vi "TestArmPathPlanner.vi"() -> ()   [LabVIEW 2017]
uses:
  General/PathPlanning/TypeDefs/Point2D.ctl
  General/MotionProfiling/TypeDefs/MotionProfileGeneratorParams.ctl
  <vilib>/Rock Robotics/WPI/ThirdParty/Phoenix-LabVIEW/Motor Controller/Controls/CTRE_Phoenix_MotorControl_TrajectoryPointTimeDur.ctl
  General/MotionProfiling/TypeDefs/TrajectoryPoint.ctl
panel:
  out "Arm Rotation":T1(graph)
  out "Arm Extension":T1(graph)
  out "Overall Motion":T1(graph)
  out "TravelTime (s)":dbl
  in  "MotionProfileGeneratorParameters":T2={"Trajectory Point Interval (ms)"=10, "Maximum Travel Speed (rpm)"=5000.0, "Velocity Ramp Time (ms)"=500.0, "Acceleration Ramp Time (ms)"=200.0} {"Acceleration Ramp Time (ms)" min=1.0; "Velocity Ramp Time (ms)" min=1.0; "Maximum Travel Speed (rpm)" min=0.0; "Trajectory Point Interval (ms)" items=["TrajectoryDuration_0ms"=0, "TrajectoryDuration_5ms"=5, "TrajectoryDuration_10ms"=10, "TrajectoryDuration_20ms"=20, "TrajectoryDuration_30ms"=30, "TrajectoryDuration_40ms"=40, "TrajectoryDuration_50ms"=50, "TrajectoryDuration_100ms"=100]}
  in  "EndPoint":T4={"X"=30.0, "Y"=30.0}
  in  "StartPoint":T4={"X"=30.0, "Y"=-24.0}
  in  "PathPointSpacing (in)":dbl=0.25
  in  "MaxArmLength":dbl=48.0
  in  "MinArmLength":dbl=24.0
  out "PathLength (in)":dbl
  out "NumPoints":i32
  out "Path":cluster{dbl[], dbl[]}[](graph)
  out "Update Rate (Hz)":dbl
  in  "stop":bool
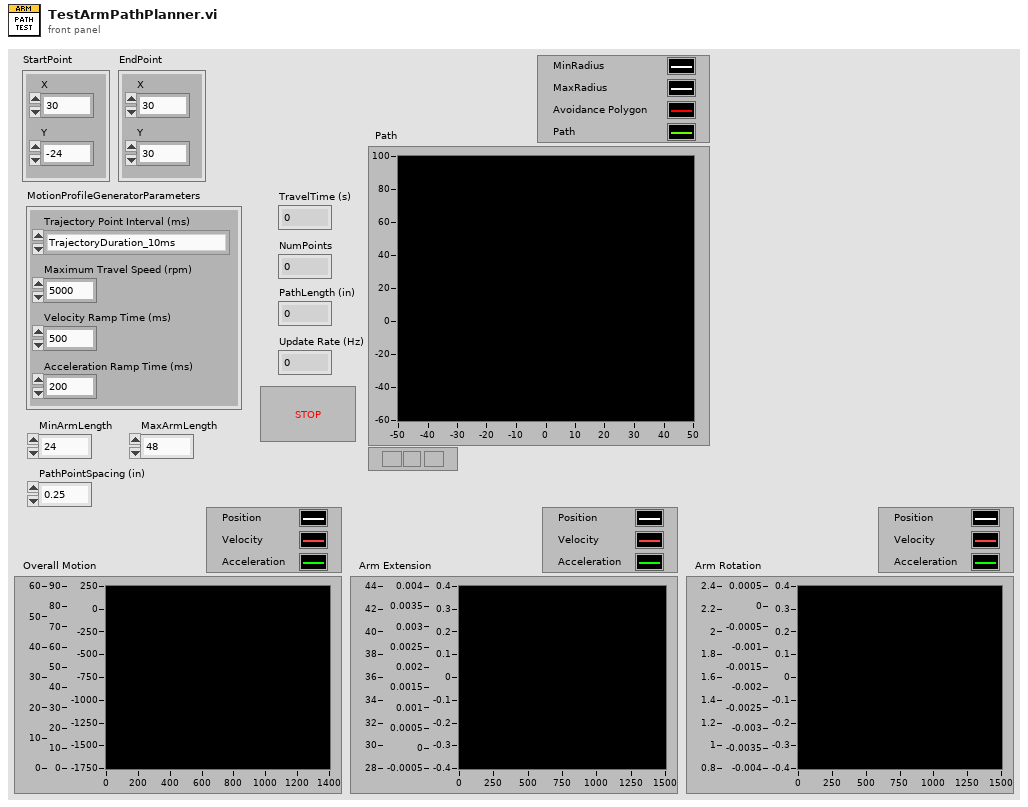
[diagram p1: front panel]
types:
  T1 = cluster{dbl, "Trajectory Point Interval (ms)":i32, dbl[][]}
  T2 = typedef "MotionProfileGeneratorParams.ctl" = cluster{"Trajectory Point Interval (ms)":T3, "Maximum Travel Speed (rpm)":dbl, "Velocity Ramp Time (ms)":dbl, "Acceleration Ramp Time (ms)":dbl}
  T3 = typedef "CTRE_Phoenix_MotorControl_TrajectoryPointTimeDur.ctl" = i32
  T4 = typedef "Point2D.ctl" = cluster{"X":dbl, "Y":dbl}
  T5 = typedef "TrajectoryPoint.ctl" = cluster{"Position ":dbl, "Velocity ":dbl, "Time (ms)":T3, "Last Point":bool}
  T6 = typedef "ArmCoordinate.ctl" = cluster{"Radius (in)":dbl, "Angle (rad)":dbl}
  T7 = cluster{dbl, "Trajectory Point Interval (ms)":T3, dbl[][]}
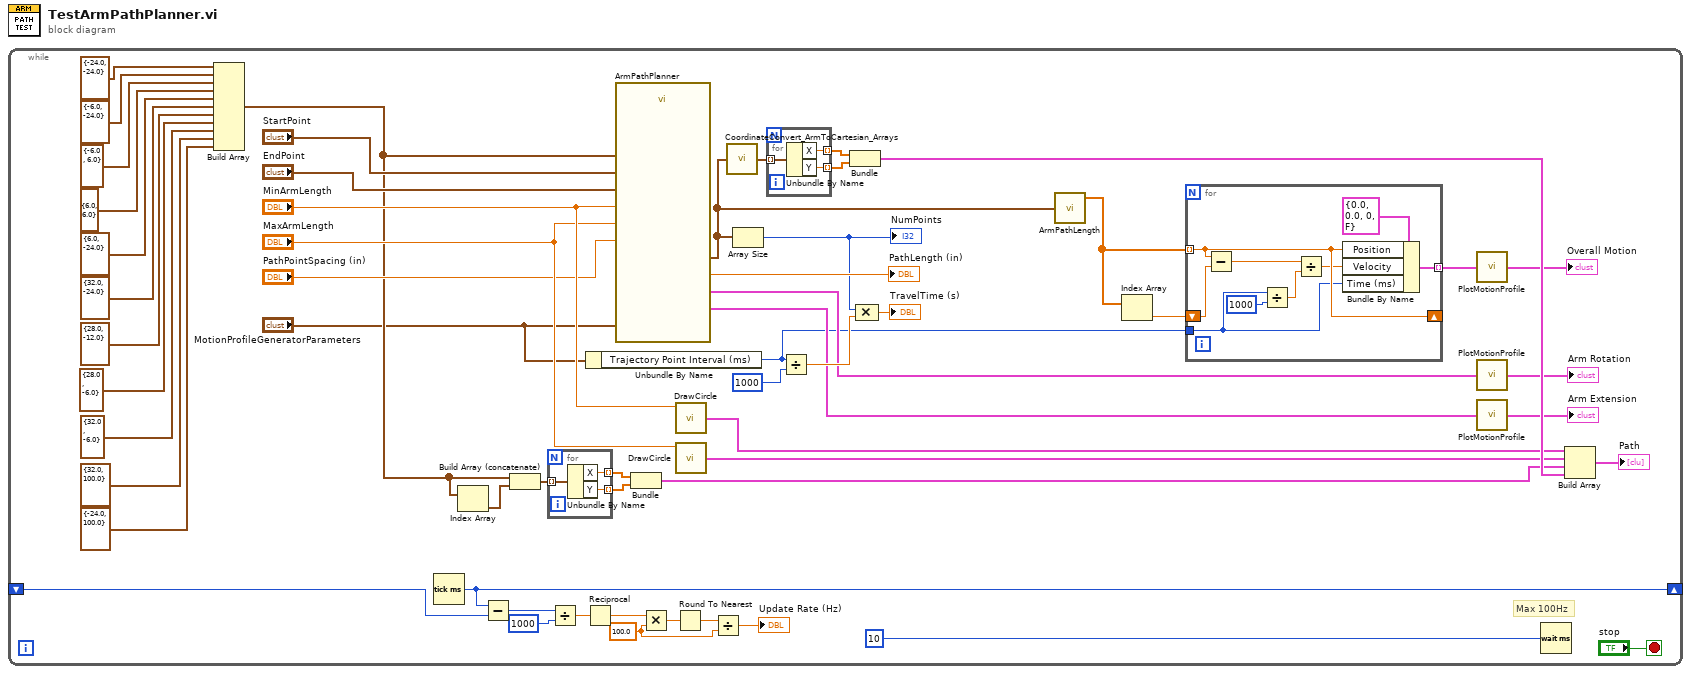
[diagram p0: block diagram]
diagram:
  n1 = while {
    shift-right: [w47] -> _
    shift-left: _ -> [w48]
    stop <- "stop" stop-if-true
    w50 = 100.0 ("y")
    # "Max 100Hz"
    n2 = Build Array(T4 {"X"=-24.0, "Y"=-24.0} ("2DPoint"), T4 {"X"=-6.0, "Y"=-24.0} ("2DPoint"), T4 {"X"=-6.0, "Y"=6.0} ("2DPoint"), T4 {"X"=6.0, "Y"=6.0} ("2DPoint"), T4 {"X"=6.0, "Y"=-24.0} ("2DPoint"), T4 {"X"=32.0, "Y"=-24.0} ("2DPoint"), T4 {"X"=28.0, "Y"=-12.0} ("2DPoint"), T4 {"X"=28.0, "Y"=-6.0} ("2DPoint"), T4 {"X"=32.0, "Y"=-6.0} ("2DPoint"), T4 {"X"=32.0, "Y"=100.0} ("2DPoint"), T4 {"X"=-24.0, "Y"=100.0} ("2DPoint")) -> (w16:T4[])
    n3 = Tick Count (ms)() -> (millisecond timer value=w47:u32)
    n4 = Index Array(array=w16) -> (element=w22:T4)  [unwired: 1 in]
    n5 = Subtract(x=w47, y=w48) -> (x-y=w56:u32)
    n6 = Build Array (concatenate)(w16, w22) -> (w23:T4[])
    n7 = for {
      tunnel: w23 -> [w69] mode=indexing
      tunnel: [w68] -> w38 mode=indexing
      tunnel: [w67] -> w39 mode=indexing
      n8 = Unbundle By Name(w69) -> ("X"=w68:dbl, "Y"=w67:dbl)
    }
    n9 = Divide(x=w56, y=u32 1000) -> (x/y=w54:dbl)
    n10 = Reciprocal(x=w54) -> (1/x=w53:dbl)
    n11 = Unbundle By Name("MotionProfileGeneratorParameters") -> ("Trajectory Point Interval (ms)"=w3:T3)
    n12 = call "ArmPathPlanner.vi"("StartPoint"="StartPoint", "EndPoint"="EndPoint", "PathPointSpacing (in)"="PathPointSpacing (in)", "MinArmLength"="MinArmLength", "MaxArmLength"="MaxArmLength", "AvoidancePolygon"=w16, "MotionProfileGeneratorParameters"="MotionProfileGeneratorParameters") -> ("Path"=w4:T6[], "RotatePath"=w8:T5[], "ExtendPath"=w7:T5[], "PathLength (in)"=→"PathLength (in)":dbl)  [unwired: 9 in]
    n13 = Bundle(w38, w39) -> (w37:cluster{dbl[], dbl[]})  [unwired: 1 in]
    n14 = Multiply(x=w53, y=w50) -> (x*y=w52:dbl)
    n15 = Round To Nearest(number=w52) -> (nearest integer value=w51:dbl)
    n16 = call "DrawCircle.vi"("Radius"="MinArmLength") -> ("Points"=w35:cluster{"X":dbl[], "Y":dbl[]})  [unwired: 3 in]
    n17 = call "DrawCircle.vi"("Radius"="MaxArmLength") -> ("Points"=w33:cluster{"X":dbl[], "Y":dbl[]})  [unwired: 3 in]
    n18 = Divide(x=w51, y=w50) -> (x/y=→"Update Rate (Hz)":dbl)
    n19 = call "CoordinateConvert_ArmToCartesian_Arrays.vi"("ArmCoordinates"=w4) -> ("XYPoints"=w44:T4[])
    n20 = Array Size(array=w4) -> (size(s)=w13:i32)
    "NumPoints" <- w13
    n21 = for {
      tunnel: w44 -> [w72] mode=indexing
      tunnel: [w71] -> w43 mode=indexing
      tunnel: [w70] -> w42 mode=indexing
      n22 = Unbundle By Name(w72) -> ("X"=w71:dbl, "Y"=w70:dbl)
    }
    n23 = Divide(x=w3, y=1000) -> (x/y=w11:dbl)
    n24 = Bundle(w43, w42) -> (w40:cluster{dbl[], dbl[]})  [unwired: 1 in]
    n25 = Compound Arithmetic op=MULTIPLY(w13, w11) -> (→"TravelTime (s)":dbl)
    n26 = call "ArmPathLength.vi"("ArmPathIn"=w4) -> ("IndexedPathLength"=w2:dbl[])  [unwired: 2 in, 2 out]
    n27 = Index Array(array=w2) -> (element=w1:dbl)  [unwired: 1 in]
    n28 = for {
      tunnel: [w65] -> w5 mode=indexing
      tunnel: w2 -> [w64] mode=indexing
      tunnel: w3 -> [w62]
      shift-right: [w64] -> _
      shift-left: w1 -> [w63]
      n29 = Subtract(x=w64, y=w63) -> (x-y=w60:dbl)
      n30 = Divide(x=w62, y=1000) -> (x/y=w59:dbl)
      n31 = Divide(x=w60, y=w59) -> (x/y=w58:dbl)
      n32 = Bundle By Name(cluster=T5 {"Position "=0.0, "Velocity "=0.0, "Time (ms)"=0, "Last Point"=FALSE} ("trajectory point"), "Position"=w64, "Velocity"=w58, "Time (ms)"=w62) -> (w65:T5)
    }
    n33 = call "PlotMotionProfile.vi"("Trajectory Points"=w5) -> ("MotionProfileGraph"=→"Overall Motion":T7)
    n34 = call "PlotMotionProfile.vi"("Trajectory Points"=w8) -> ("MotionProfileGraph"=→"Arm Rotation":T7)
    n35 = call "PlotMotionProfile.vi"("Trajectory Points"=w7) -> ("MotionProfileGraph"=→"Arm Extension":T7)
    n36 = Wait (ms)(milliseconds to wait=u32 10) -> ()  [unwired: 1 out]
    n37 = Build Array(w35, w33, w37, w40) -> (→"Path":cluster{"X":dbl[], "Y":dbl[]}[])
  }
